vi "Offset Async Buffers.vi"(8 "error in (no error)":errorcluster, 11 "Framework in":refnum<class "Framework.lvclass">) -> (0 "error out":errorcluster, 3 "Framework out":refnum<class "Framework.lvclass">)   [LabVIEW 2017, in "DSF Core.lvlib" / "Framework.lvclass"]
uses:
  Framework.lvclass
  Framework.lvclass/Framework.ctl
  Buffers/Buffers.lvclass/Buffers.ctl
  Interfaces/Dispatcher/Inline Buffer Parameters.ctl
  Buffer/Buffer.lvclass
  C:/Git/DSF/LabVIEW-Memory/Source/Classes/Pointer/Pointer.lvclass
  Buffers/Buffers.lvclass
  LabVIEW-Memory/Source/Classes/Pointer/Pointer.lvclass
  Interfaces/Dispatcher/Dispatcher Interface.lvclass
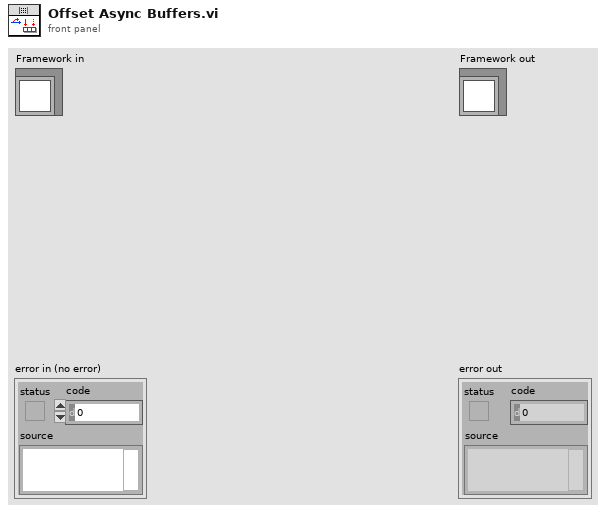
[diagram p1: front panel]
types:
  T1 = typedef "DSF Core.lvlib/Dispatcher Interface.lvclass/Inline Buffer Parameters.ctl" = cluster{"address":u64, "size":u64}
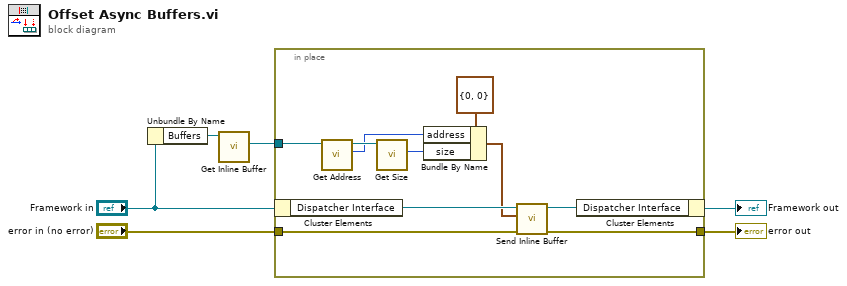
[diagram p0: block diagram]
diagram:
  n1 = Unbundle By Name("Framework in") -> ("Buffers"=w2:refnum<class "Buffers.lvclass">)
  n2 = call "Get Inline Buffer.vi"("Buffers in"=w2) -> ("Inline Buffer"=w1:refnum<class "Buffer.lvclass">)  [unwired: 9 in, 1 out]
  n3 = in-place {
    in-place-border: w1 -> [w16]
    in-place-border: "error in (no error)" -> [w13]
    in-place-border: [w8] -> w5
    n4 = in-place-cluster #1("Framework in") -> ("Dispatcher Interface"=w14:refnum<class "Dispatcher Interface.lvclass">)
    n5 = call "Get Address.vi"("Pointer in"=w16) -> ("address"=w10:u64, "Pointer out"=w15:refnum<class "Buffer.lvclass">)  [unwired: 9 in]
    n6 = call "Get Size.vi"("Pointer in"=w15) -> ("size"=w11:u64)  [unwired: 9 in, 1 out]
    n7 = Bundle By Name(cluster=T1 {"address"=0, "size"=0} ("Inline Buffer Parameters"), "address"=w10, "size"=w11) -> (w7:T1)
    n8 = call "Send Inline Buffer.vi"("error in (no error)"=w13, "Inline Buffer Parameters"=w7, "Dispatcher Interface in"=w14) -> ("error out"=w8:errorcluster, "Dispatcher Interface out"=w9:refnum<class "Dispatcher Interface.lvclass">)  [unwired: 7 in]
    n9 = in-place-cluster #1("Dispatcher Interface"=w9) -> (→"Framework out":refnum<class "Framework.lvclass">)
  }
  "error out" <- w5
